vi "Write Single Coil.vi"(8 "error in (no error)":errorcluster, 9 "coil value":bool, 10 "address":u16, 11 "device data model in":refnum<class "ICPCON ET Data Model.lvclass">) -> (0 "error out":errorcluster, 3 "device data model out":refnum<class "ICPCON ET Data Model.lvclass">)   [LabVIEW 2021, in "ICPCON ET Data Model.lvclass"]
doc: "Writes the value of a single coil."
uses:
  ICPCON ET Data Model.lvclass
  ICPCON ET Data Model.lvclass/ICPCON ET Data Model.ctl
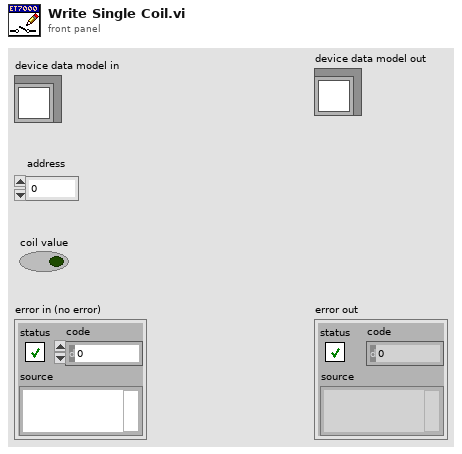
[diagram p1: front panel]
types:
  T1 = typedef "ICPCON ET Data Model.lvclass/Data Model.ctl" = cluster{"UTC":u64, "DI":bool[], "DO":bool[], "IR":u16[], "HR":u16[], "ES":u8}
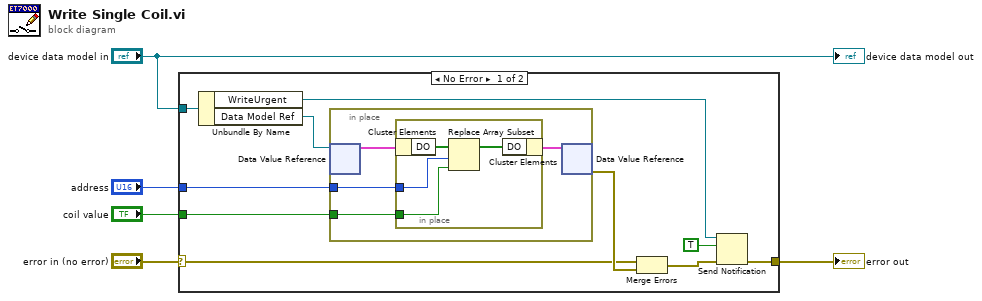
[diagram p0: block diagram]
diagram:
  n1 = case shown="No Error" "error in (no error)" {
    selector: "error in (no error)" -> [w10 w24]
    tunnel: "device data model in" -> [w15 _]
    tunnel: [w7 w24] -> w1
    tunnel: "address" -> [w14 _]
    tunnel: "coil value" -> [w13 _]
    frame No Error {
      n2 = Unbundle By Name(w15) -> ("WriteUrgent"=w6:refnum<notifier>, "Data Model Ref"=w12:refnum<data-value>)
      n3 = in-place {
        in-place-border: w14 -> [w19]
        in-place-border: w13 -> [w18]
        n4 = in-place-dvr #1(w12) -> (w17:T1)  [unwired: 1 out]
        n5 = in-place {
          in-place-border: w19 -> [w23]
          in-place-border: w18 -> [w22]
          n6 = in-place-cluster #2(w17) -> ("DO"=w21:bool[])
          n7 = Replace Array Subset(array=w21, new element=w22, index=w23) -> (w20:bool[])
          n8 = in-place-cluster #2("DO"=w20) -> (w16:T1)
        }
        n9 = in-place-dvr #1(w16) -> (w11:errorcluster)  [unwired: 1 out]
      }
      n10 = Merge Errors(w10, w11) -> (w8:errorcluster)
      n11 = Send Notification(notification=TRUE, notifier=w6, error in (no error)=w8) -> (error out=w7:errorcluster)  [unwired: 1 out]
    }
    frame Error {
    }
  }
  "error out" <- w1
  "device data model out" <- "device data model in"
